vi "maintainVideoBuffer.vi"(8 "error in (no error)":errorcluster, 9 "Video buffer size (frames)":i32, 10 "Image pointer recycling queue":refnum<queue>, 11 "Video queue":refnum<queue>) -> (0 "error out":errorcluster)   [LabVIEW 2017]
doc: "Maintain the # of elements in the video queue to be less than the desired size of the buffer, and recycle the image pointers to be reused when removed from the buffer."
uses:
  <vilib>/vision/Image Controls.llb/IMAQ Image.ctl
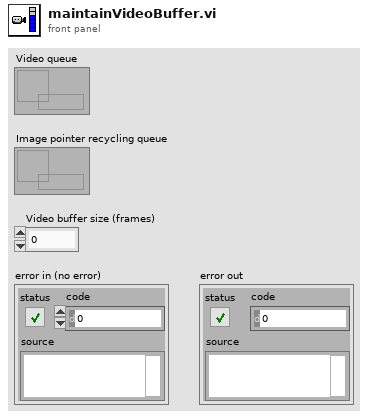
[diagram p1: front panel]
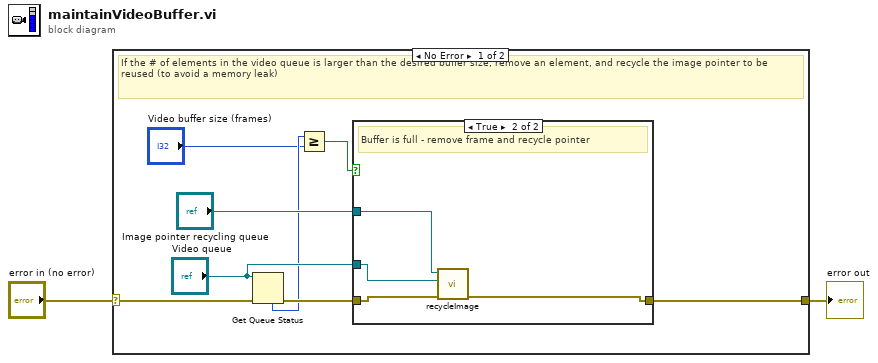
[diagram p0: block diagram]
diagram:
  n1 = case shown="No Error" "error in (no error)" {
    selector: "error in (no error)" -> [w3 w16]
    tunnel: [w9 w16] -> w2
    frame No Error {
      # "If the # of elements in the video queue is larger than the desired buffer size, remove an element, and recycle the image pointer to be reused (to avoid a memory leak)"
      n2 = Get Queue Status(queue="Video queue", error in (no error)=w3) -> (error out=w8:errorcluster, # elements in queue=w5:i32)  [unwired: 1 in, 6 out]
      n3 = Greater Or Equal?(x=w5, y="Video buffer size (frames)") -> (x >= y?=w6:bool)
      n4 = case shown="True" w6 {
        tunnel: "Video queue" -> [_ w15]
        tunnel: w8 -> [w11 w14]
        tunnel: [w11 w12] -> w9
        tunnel: "Image pointer recycling queue" -> [_ w13]
        frame False {
          # "Buffer not full yet"
        }
        frame True {
          # "Buffer is full - remove frame and recycle pointer"
          n5 = call "recycleImage.vi"("error in (no error)"=w14, "Video queue"=w15, "Image pointer recylcing queue"=w13) -> ("error out"=w12:errorcluster)  [unwired: 8 in]
        }
      }
    }
    frame Error {
    }
  }
  "error out" <- w2
